vi "Remove TypeDef from Cluster.vi"(7 "configuration 1.4":T1={"plugins"=[{"core"={"name"="", "components"=[], "cycle timing"={"priority"=10000, "decimation"=1, "offset"=0}}, "component settings"=[], "threads"=[{"core"={"processor"=-2, "priority offset"=0}, "component settings"=[], "transfer groups"=[{"core"={"name"="Group", "direction"=0, "cycle timing"={"priority"=100, "decimation"=1, "offset"=0}, "timeout behavior"=0, "enable conversion"=FALSE}, "component settings"=[], "transfers"=[{"core"={"name"="Transfer"}, "component settings"=[], "channels"=[{"core"={"name"="Channel", "units"="V", "engine data type"=2, "string data type"=2, "string offset"=0}, "component settings"=[]}]}]}]}]}]}) -> (8 "JSON string":string)   [LabVIEW 2023]
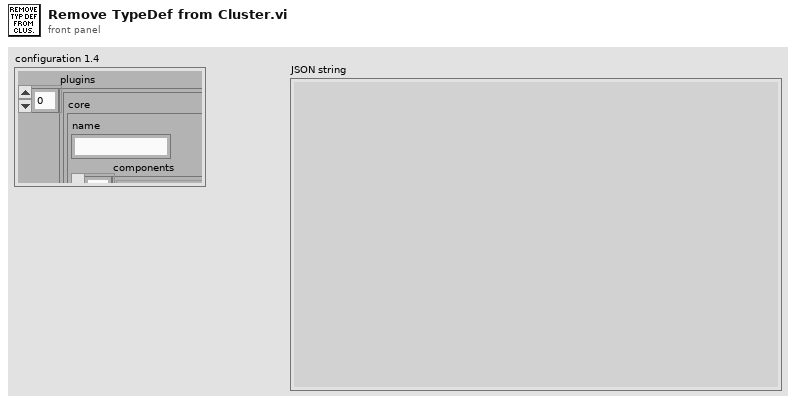
[diagram p1: front panel]
types:
  T1 = cluster{"plugins":cluster{"core":cluster{"name":string, "components":string[], "cycle timing":cluster{"priority":u64, "decimation":u64, "offset":u64}}, "component settings":cluster{"component":string, "values":cluster{"key":string, "value":string}[]}[], "threads":cluster{"core":cluster{"processor":i32, "priority offset":i16}, "component settings":cluster{"component":string, "values":cluster{"key":string, "value":string}[]}[], "transfer groups":cluster{"core":cluster{"name":string, "direction":i32, "cycle timing":cluster{"priority":u64, "decimation":u64, "offset":u64}, "timeout behavior":u8, "enable conversion":bool}, "component settings":cluster{"component":string, "values":cluster{"key":string, "value":string}[]}[], "transfers":cluster{"core":cluster{"name":string}, "component settings":cluster{"component":string, "values":cluster{"key":string, "value":string}[]}[], "channels":cluster{"core":cluster{"name":string, "units":string, "engine data type":u8, "string data type":u8, "string offset":u64}, "component settings":cluster{"component":string, "values":cluster{"key":string, "value":string}[]}[]}[]}[]}[]}[]}[]}
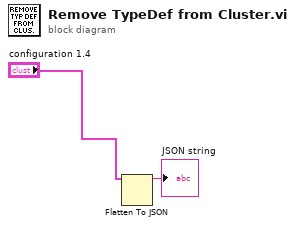
[diagram p0: block diagram]
diagram:
  n1 = Flatten To JSON(anything="configuration 1.4") -> (JSON string=→"JSON string":string)  [unwired: 2 in, 1 out]
